vi "getNsamples.vi"(8 "error in (no error)":errorcluster, 11 "params":refnum<class "JSON Value.lvclass">) -> (0 "error out":errorcluster, 3 "data":refnum<class "JSON Value.lvclass">)   [LabVIEW 2017]
uses:
  <vilib>/NI/JSON Support for LabVIEW/JSON Value/JSON Value.lvclass
  <vilib>/NI/JSON Support for LabVIEW/JSON Value/Object/Get Value/Get Value (Numeric).vi
  <vilib>/NI/JSON Support for LabVIEW/JSON Value/Object/Get Value/Get Value (Value).vi
  <vilib>/NI/JSON Support for LabVIEW/JSON Value/New JSON Value/New JSON (Numeric[]).vi
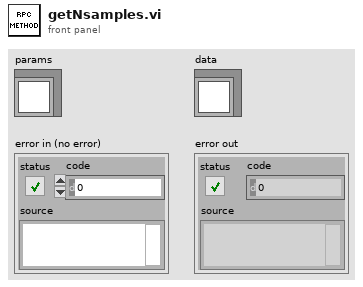
[diagram p1: front panel]
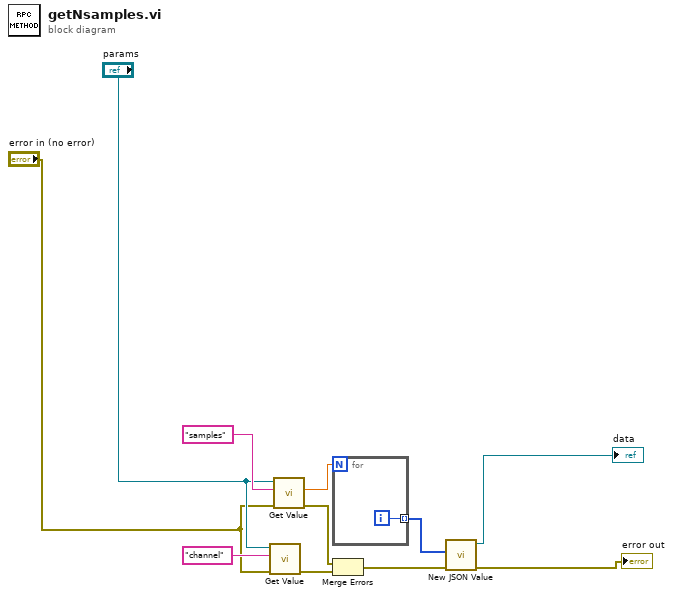
[diagram p0: block diagram]
diagram:
  n1 = call-poly <vilib>:"Get Value.vi"("error in (no error)"="error in (no error)", "key"="channel", "JSON Value in"="params") -> ("error out"=w7:errorcluster)  [unwired: 7 in, 1 out]
  n2 = call-poly <vilib>:"Get Value.vi"("error in (no error)"="error in (no error)", "key"="samples", "JSON Value in"="params") -> ("error out"=w6:errorcluster, "value"=w9:dbl)  [unwired: 7 in]
  n3 = for {
    N: w9 -> [_]
    tunnel: [w12] -> w8 mode=indexing
    i -> [w12]
  }
  n4 = Merge Errors(w6, w7) -> (w5:errorcluster)
  n5 = call-poly <vilib>:"New JSON Value.vi"("error in (no error)"=w5, "Numeric Array"=w8) -> ("error out"=→"error out":errorcluster, "JSON Value out"=→"data":refnum<class "JSON Value.lvclass">)  [unwired: 8 in]
